vi "OTP - Decode.vi"(10 "Key (Private)":string, 11 "ciphertext (Public)":string) -> (3 "original message":string)   [LabVIEW 2013]
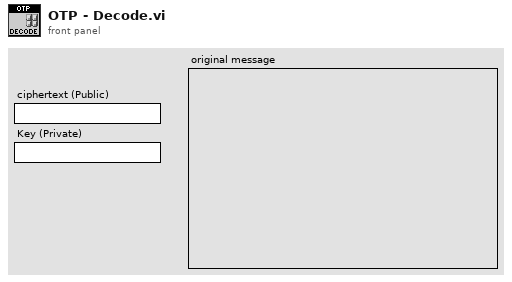
[diagram p1: front panel]
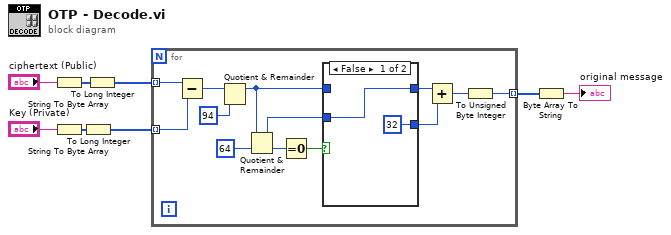
[diagram p0: block diagram]
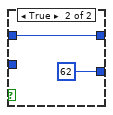
[diagram p2: hidden frame]
diagram:
  n1 = String To Byte Array(string="ciphertext (Public)") -> (unsigned byte array=w7:u8[])
  n2 = String To Byte Array(string="Key (Private)") -> (unsigned byte array=w8:u8[])
  n3 = To Long Integer(number=w8) -> (32bit integer=w4:i32[])
  n4 = To Long Integer(number=w7) -> (32bit integer=w5:i32[])
  n5 = for {
    tunnel: w4 -> [w20] mode=indexing
    tunnel: w5 -> [w21] mode=indexing
    tunnel: [w18] -> w6 mode=indexing
    n6 = Subtract(x=w21, y=w20) -> (x-y=w16:i32)
    n7 = Quotient & Remainder(x=w16, y=94) -> (x-y*floor(x/y)=w11:i32)  [unwired: 1 out]
    n8 = Quotient & Remainder(x=w11, y=64) -> (x-y*floor(x/y)=w12:i32, floor(x/y)=w14:i32)
    n9 = Equal To 0?(x=w14) -> (x = 0?=w13:bool)
    n10 = case shown="False" w13 {
      tunnel: w12 -> [w22 _]
      tunnel: w11 -> [_ w25]
      tunnel: [w22 w25] -> w10
      tunnel: [32 ("y") 62 ("y")] -> w9
      frame False {
      }
      frame True {
      }
    }
    n11 = Add(x=w10, y=w9) -> (x+y=w17:i32)
    n12 = To Unsigned Byte Integer(number=w17) -> (unsigned 8bit integer=w18:u8)
  }
  n13 = Byte Array To String(unsigned byte array=w6) -> (string=→"original message":string)
